vi "MessageQueue.vi"() -> (0 "error out":errorcluster, 3 "Queue out":refnum<queue>)   [LabVIEW 2018]
doc: "Crea la coda di messaggi per la comunicazione degli stati del controller"
uses:
  MessageCluster.ctl
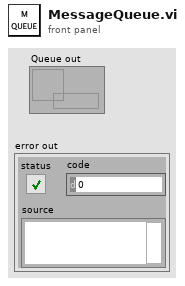
[diagram p1: front panel]
types:
  T1 = typedef "MessageCluster.ctl" = cluster{"Message":string, "Temp":i32, "Stato":enum16{"On", "Off", "Preparation", "WaitTimer", "Ready"}}
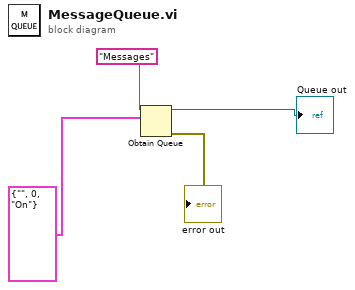
[diagram p0: block diagram]
diagram:
  n1 = Obtain Queue(name (unnamed)="Messages", element data type=T1 {"Message"="", "Temp"=0, "Stato"=enum."On"} ("Message Cluster")) -> (queue out=→"Queue out":refnum<queue>, error out=→"error out":errorcluster)  [unwired: 3 in, 1 out]
